vi "配方.vi"() -> (1 "Start_Line":string[](array[string]), 2 "End_Line":string[](array[string]))   [LabVIEW 2018]
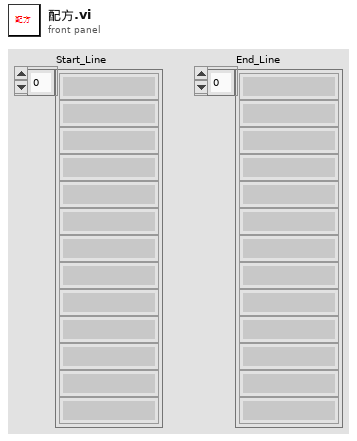
[diagram p1: front panel]
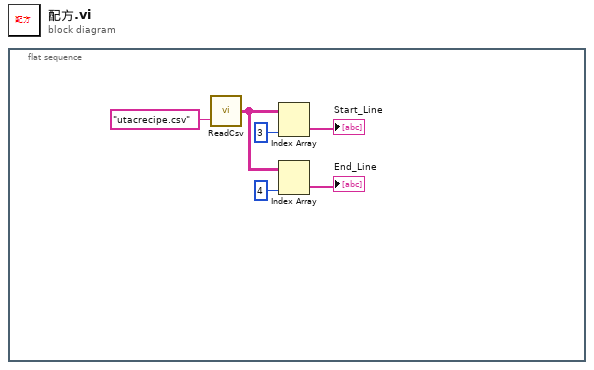
[diagram p0: block diagram]
diagram:
  n1 = flat-sequence {
    frame #0 {
      n2 = call "ReadCsv.vi"("相对路径"="utacrecipe.csv") -> ("all rows"=w4:string[][])  [unwired: 1 in]
      n3 = Index Array(array=w4, index (col)=3 ("禁用的索引 (列)")) -> (element=→"Start_Line":string[])  [unwired: 1 in]
      n4 = Index Array(array=w4, index (col)=4 ("禁用的索引 (列)")) -> (element=→"End_Line":string[])  [unwired: 1 in]
    }
  }
